vi "NH3N 随机数出数.vi"(4 "公式":cluster{"X^2":dbl, "X":dbl, "B":dbl}, 5 "测试模式":enum16{"Default", "水样测试", "零点核查", "跨度核查"}(ring), 8 "信号值原始值":dbl, 9 "原始值":dbl) -> (1 "随机数？":bool, 2 "信号值":dbl, 3 "取值输出":dbl)   [LabVIEW 2016]
uses:
  Holding Var.vi
  Process var.vi
  random number/random number.lvlib
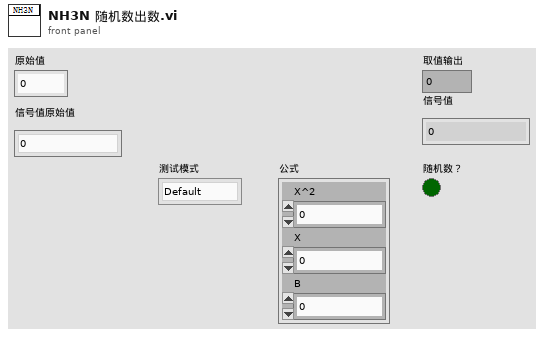
[diagram p1: front panel]
types:
  T1 = cluster{"水样参数输出":cluster{"mean":dbl, "变异系数":dbl, "随机数？":bool}, "零点参数输出":cluster{"mean":dbl, "变异系数":dbl, "随机数？":bool}, "跨度参数输出":cluster{"mean":dbl, "变异系数":dbl, "随机数？":bool}}
  T2 = cluster{"水样测试":cluster{"参数输入":cluster{"采样模式":enum16{"自动采样", "手动采样"}, "采样点数":i32, "变异系数设定值":dbl, "重新取值百分比":dbl, "偏差模式":enum16{"相对偏差", "绝对偏差"}, "相对偏差百分比":dbl, "绝对偏差值":dbl}, "采样值":dbl[], "启用":bool}, "零点核查":cluster{"参数输入":cluster{"采样模式":enum16{"自动采样", "手动采样"}, "采样点数":i32, "变异系数设定值":dbl, "重新取值百分比":dbl, "偏差模式":enum16{"相对偏差", "绝对偏差"}, "相对偏差百分比":dbl, "绝对偏差值":dbl}, "采样值":dbl[], "启用":bool}, "跨度核查":cluster{"参数输入":cluster{"采样模式":enum16{"自动采样", "手动采样"}, "采样点数":i32, "变异系数设定值":dbl, "重新取值百分比":dbl, "偏差模式":enum16{"相对偏差", "绝对偏差"}, "相对偏差百分比":dbl, "绝对偏差值":dbl}, "采样值":dbl[], "启用":bool}}
  T3 = cluster{"采样模式":enum16{"自动采样", "手动采样"}, "采样点数":i32, "变异系数设定值":dbl, "重新取值百分比":dbl, "偏差模式":enum16{"相对偏差", "绝对偏差"}, "相对偏差百分比":dbl, "绝对偏差值":dbl}
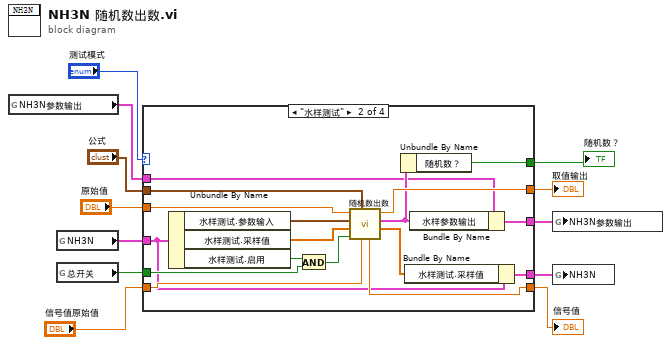
[diagram p0: block diagram]
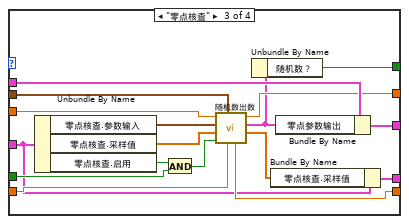
[diagram p3: hidden frame]
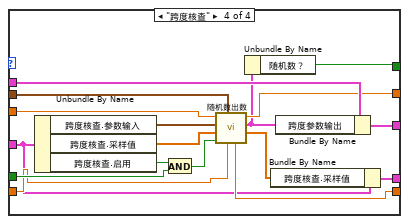
[diagram p4: hidden frame]
diagram:
  n1 = global read "Process var.vi" "NH3N参数输出"() -> (w12:T1)
  n2 = global read "Holding Var.vi" "NH3N"() -> (w3:T2)
  n3 = global read "Holding Var.vi" "总开关"() -> (w7:bool)
  n4 = case shown="\"水样测试\"" "测试模式" {
    tunnel: w3 -> [w15 w22 w37 w55]
    tunnel: w12 -> [w16 w17 w48 w65]
    tunnel: [w16 w31 w47 w64] -> w11
    tunnel: "原始值" -> [w13 w30 w46 w63]
    tunnel: [w13 w29 w45 w62] -> w8
    tunnel: w7 -> [_ w26 w44 w59]
    tunnel: "公式" -> [_ w25 w41 w58]
    tunnel: [w14 w23 w40 w56] -> w5
    tunnel: "信号值原始值" -> [w14 w24 w39 w57]
    tunnel: [w15 w21 w36 w54] -> w2
    tunnel: [_ w18 w34 w51] -> w1
    frame "Default", Default {
    }
    frame "水样测试" {
      n5 = Unbundle By Name(w22) -> ("水样测试.参数输入"=w33:T3, "水样测试.采样值"=w32:dbl[], "水样测试.启用"=w27:bool)
      n6 = And(x=w27, y=w26) -> (x .and. y?=w28:bool)
      n7 = call "随机数出数.vi"("信号值原始值"=w24, "公式"=w25, "启用"=w28, "采样值"=w32, "参数输入"=w33, "监测值原始值"=w30) -> ("采样值输出"=w20:dbl[], "参数输出"=w19:cluster{"mean":dbl, "变异系数":dbl, "随机数？":bool}, "取值输出"=w29:dbl, "信号值"=w23:dbl)  [unwired: 2 in]
      n8 = Unbundle By Name(w19) -> ("随机数？"=w18:bool)
      n9 = Bundle By Name(cluster=w22, "水样测试.采样值"=w20) -> (w21:T2)
      n10 = Bundle By Name(cluster=w17, "水样参数输出"=w19) -> (w31:T1)
    }
    frame "零点核查" {
      n11 = Unbundle By Name(w37) -> ("零点核查.参数输入"=w50:T3, "零点核查.采样值"=w49:dbl[], "零点核查.启用"=w43:bool)
      n12 = And(x=w43, y=w44) -> (x .and. y?=w42:bool)
      n13 = call "随机数出数.vi"("信号值原始值"=w39, "公式"=w41, "启用"=w42, "采样值"=w49, "参数输入"=w50, "监测值原始值"=w46) -> ("采样值输出"=w38:dbl[], "参数输出"=w35:cluster{"mean":dbl, "变异系数":dbl, "随机数？":bool}, "取值输出"=w45:dbl, "信号值"=w40:dbl)  [unwired: 2 in]
      n14 = Unbundle By Name(w35) -> ("随机数？"=w34:bool)
      n15 = Bundle By Name(cluster=w37, "零点核查.采样值"=w38) -> (w36:T2)
      n16 = Bundle By Name(cluster=w48, "零点参数输出"=w35) -> (w47:T1)
    }
    frame "跨度核查" {
      n17 = Unbundle By Name(w55) -> ("跨度核查.参数输入"=w67:T3, "跨度核查.采样值"=w66:dbl[], "跨度核查.启用"=w60:bool)
      n18 = And(x=w60, y=w59) -> (x .and. y?=w61:bool)
      n19 = call "随机数出数.vi"("信号值原始值"=w57, "公式"=w58, "启用"=w61, "采样值"=w66, "参数输入"=w67, "监测值原始值"=w63) -> ("采样值输出"=w53:dbl[], "参数输出"=w52:cluster{"mean":dbl, "变异系数":dbl, "随机数？":bool}, "取值输出"=w62:dbl, "信号值"=w56:dbl)  [unwired: 2 in]
      n20 = Unbundle By Name(w52) -> ("随机数？"=w51:bool)
      n21 = Bundle By Name(cluster=w55, "跨度核查.采样值"=w53) -> (w54:T2)
      n22 = Bundle By Name(cluster=w65, "跨度参数输出"=w52) -> (w64:T1)
    }
  }
  "取值输出" <- w8
  "信号值" <- w5
  "随机数？" <- w1
  n23 = global write "Process var.vi" "NH3N参数输出"(w11) -> ()
  n24 = global write "Holding Var.vi" "NH3N"(w2) -> ()
